vi "tcsOfc_logEvent_degreeOfFreedom.vi"(8 "error in (no error)":errorcluster, 11 "logevent_degreeOfFreedom_Ctl":T1={"dof[50]"=[0.0, 0.0, 0.0, 0.0, 0.0, 0.0, 0.0, 0.0, 0.0, 0.0, 0.0, 0.0, 0.0, 0.0, 0.0, 0.0, 0.0, 0.0, 0.0, 0.0, 0.0, 0.0, 0.0, 0.0, 0.0, 0.0, 0.0, 0.0, 0.0, 0.0, 0.0, 0.0, 0.0, 0.0, 0.0, 0.0, 0.0, 0.0, 0.0, 0.0, 0.0, 0.0, 0.0, 0.0, 0.0, 0.0, 0.0, 0.0, 0.0, 0.0], "timestamp"=0.0, "priority"=0}) -> (0 "error out":errorcluster, 2 "function return":i32, 3 "logevent_degreeOfFreedom_Ctl out":T1)   [LabVIEW 2016, in "SALLV_tcsOfc.lvlib"]
doc: "int tcsOfc_shm_logEvent_degreeOfFreedomLV(tcsOfc_logevent_degreeOfFreedomLV *logevent_degreeOfFreedom_Ctl );"
uses:
  SALLV_tcsOfc.lvlib
  DataTypes/logevent_degreeOfFreedom.ctl
  SALLV_tcsOfc.so
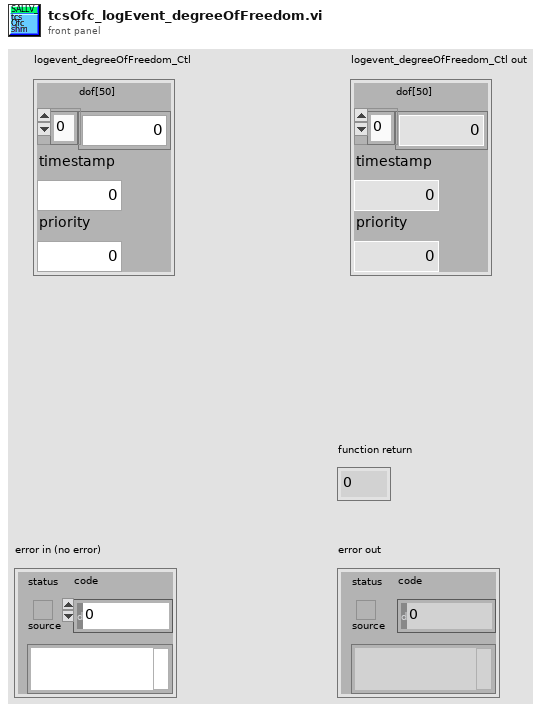
[diagram p1: front panel]
types:
  T1 = typedef "SALLV_tcsOfc.lvlib/logevent_degreeOfFreedom.ctl" = cluster{"dof[50]":dbl[], "timestamp":dbl, "priority":i32}
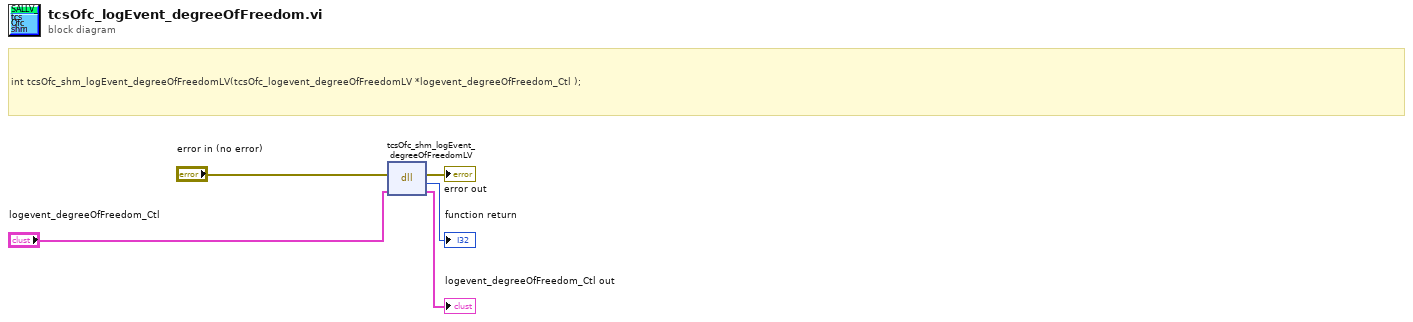
[diagram p0: block diagram]
diagram:
  # "int tcsOfc_shm_logEvent_degreeOfFreedomLV(tcsOfc_logevent_degreeOfFreedomLV *logevent_degreeOfFreedom_Ctl );"
  n1 = dll-call lib="home/ttsai/Documents/salAPI/SALLV_tcsOfc/SALLV_tcsOfc.*" fn="tcsOfc_shm_logEvent_degreeOfFreedomLV"(error in="error in (no error)", "logevent_degreeOfFreedom_Ctl"="logevent_degreeOfFreedom_Ctl") -> (error out=→"error out":errorcluster, →"function return":i32, "logevent_degreeOfFreedom_Ctl"=→"logevent_degreeOfFreedom_Ctl out":T1)  [unwired: 2 in, 1 out]
